vi "DriveModuleControl.vi"(8 "error in":errorcluster, 9 "Actual State":T1={"Speed"=0.0, "Angle"={"VALUE"=0.0, "COS"=1.0, "SIN"=0.0}} {"Angle"."SIN" format="%13.4f"; "Angle"."COS" format="%13.4f"; "Angle"."VALUE" format="%13.4f"}, 10 "Desired State":T1={"Speed"=0.0, "Angle"={"VALUE"=0.0, "COS"=1.0, "SIN"=0.0}} {"Angle"."SIN" format="%13.4f"; "Angle"."COS" format="%13.4f"; "Angle"."VALUE" format="%13.4f"}, 11 "ModualNamePrefix":i32) -> (0 "error out":errorcluster)   [LabVIEW 2023]
uses:
  <vilib>/Rock Robotics/WPI/ThirdParty/JAS_Junk/TrajLib/TypeDef/SWERVE_DRIVE_MODULE_STATE.ctl
  <vilib>/Rock Robotics/WPI/ThirdParty/JAS_Junk/TrajLib/TypeDef/ROTATION2D.ctl
  <vilib>/Rock Robotics/WPI/ThirdParty/JAS_Junk/TrajLib/Rotation2d_Minus.vi
  <vilib>/Rock Robotics/WPI/ThirdParty/JAS_Junk/TrajLib/Rotation2d_GetRadians.vi
  <vilib>/Rock Robotics/WPI/ThirdParty/JAS_Junk/TrajLib/SwerveModuleState_New.vi
  <vilib>/Rock Robotics/WPI/ThirdParty/JAS_Junk/TrajLib/Rotation2d_RotateBy.vi
  <vilib>/Rock Robotics/WPI/ThirdParty/JAS_Junk/TrajLib/Rotation2d_CreateAngle.vi
  <vilib>/Rock Robotics/WPI/ThirdParty/JAS_Junk/TrajLib/SimpleMotorFF_Calculate.vi
  <vilib>/Rock Robotics/WPI/ThirdParty/JAS_Junk/TrajLib/PIDController_AtSetpoint.vi
  <vilib>/Rock Robotics/WPI/ThirdParty/JAS_Junk/TrajLib/PIDController_SetPIDF.vi
  <vilib>/Rock Robotics/WPI/ThirdParty/JAS_Junk/TrajLib/PIDController_SetDerivativeFilter.vi
  <vilib>/Rock Robotics/WPI/ThirdParty/JAS_Junk/TrajLib/PIDController_SetIntegratorRange.vi
  <vilib>/Rock Robotics/WPI/ThirdParty/JAS_Junk/TrajLib/PIDController_SetTolerancePandV.vi
  <vilib>/Rock Robotics/WPI/ThirdParty/JAS_Junk/TrajLib/PIDController_DisableContinousInput.vi
  <vilib>/Rock Robotics/WPI/ThirdParty/JAS_Junk/TrajLib/PIDController_EnableContinousInput.vi
  <vilib>/Rock Robotics/WPI/ThirdParty/JAS_Junk/TrajLib/PIDController_Reset.vi
  <vilib>/Rock Robotics/WPI/ThirdParty/JAS_Junk/TrajLib/PIDController_New.vi
  <vilib>/Rock Robotics/WPI/ThirdParty/JAS_Junk/TrajLib/PIDController_SetOutputLimits.vi
  <vilib>/Rock Robotics/WPI/ThirdParty/JAS_Junk/TrajLib/VI/PIDController_SetIntegratorZone.vi
  <vilib>/Rock Robotics/WPI/ThirdParty/JAS_Junk/TrajLib/SlewRateLimiter_New.vi
  <vilib>/Rock Robotics/WPI/ThirdParty/JAS_Junk/TrajLib/SlewRateLimiter_Reset.vi
  <vilib>/Rock Robotics/WPI/ThirdParty/JAS_Junk/TrajLib/SlewRateLimiter_Calculate.vi
  <vilib>/Rock Robotics/WPI/ThirdParty/JAS_Junk/TrajLib/SlewRateLimiter_SetRate.vi
  <vilib>/Rock Robotics/WPI/ThirdParty/JAS_Junk/TrajLib/Rotation2d_UnaryMinus.vi
  <vilib>/Rock Robotics/WPI/ThirdParty/JAS_Junk/TrajLib/Rotation2d_CreateXY.vi
  <vilib>/Rock Robotics/WPI/ThirdParty/JAS_Junk/TrajLib/PIDController_NewPeriod.vi
  <vilib>/Rock Robotics/WPI/ThirdParty/JAS_Junk/TrajLib/Util_GetTime.vi
  <vilib>/Rock Robotics/WPI/ThirdParty/JAS_Junk/TrajLib/Util_CalcDist.vi
  <vilib>/Rock Robotics/SystemInterfaces/NetworkCommunication/NetComm_UsageReport_report.vi
  <vilib>/Rock Robotics/WPI/ThirdParty/JAS_Junk/TrajLib/VI/Util_GetTime_U32.vi
  DriveGlobal.vi
  <vilib>/Rock Robotics/SystemInterfaces/Utilities/FPGA_UtilitiesRead LocalTime.vi
  <vilib>/Rock Robotics/WPI/ThirdParty/JAS_Junk/TrajLib/VI/Util_GetTime_U64.vi
  <vilib>/Rock Robotics/WPI/ThirdParty/JAS_Junk/TrajLib/Globals/Util_LibraryGlobals.vi
  <vilib>/Rock Robotics/WPI/ThirdParty/JAS_Junk/TrajLib/PIDController_AdvCalculate_FF_Sp_Pv.vi
  <vilib>/Rock Robotics/Network Tables/NT Write Number.vi
  <vilib>/Rock Robotics/WPI/ThirdParty/JAS_Junk/TrajLib/Trajectory_Library.lvlib
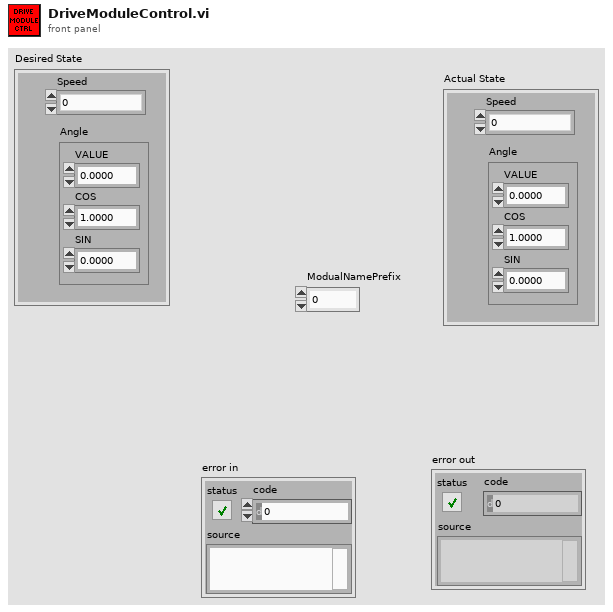
[diagram p1: front panel]
types:
  T1 = typedef "Trajectory_Library.lvlib/SWERVE_DRIVE_MODULE_STATE.ctl" = cluster{"Speed":dbl, "Angle":T2}
  T2 = typedef "Trajectory_Library.lvlib/ROTATION2D.ctl" = cluster{"VALUE":dbl, "COS":dbl, "SIN":dbl}
  T3 = typedef "Trajectory_Library.lvlib/SIMPLE_MOTOR_FF.ctl" = cluster{"Ks":dbl, "Kv":dbl, "Ka":dbl, "KnInv":dbl}
  T4 = typedef "Trajectory_Library.lvlib/PID_ADV_LIMITS.ctl" = cluster{"MaxInput":dbl, "MinInput":dbl, "Continuous":bool, "MaxOutput":dbl, "MinOutput":dbl}
  T5 = typedef "Trajectory_Library.lvlib/PID_ADV_TUNING.ctl" = cluster{"Kf":dbl, "Kp":dbl, "Ki":dbl, "Kd":dbl, "MaximumIntegral":dbl, "MinimumIntegral":dbl, "Filter Derivative":bool, "IntegralZone":dbl}
  T6 = typedef "WPI_MotorControlDeviceRef.ctl" = cluster{"DeviceStatus":errorcluster, "Type":T7, "PWM":cluster{"PWM Channel":T8, "DeadBand":T9}, "CAN":cluster{"Device Number":u8, "SetOutput VI Ref":variant, "GetOutput VI Ref":variant, "Enable VI Ref":variant, "Disable VI Ref":variant, "Data":variant}, "Invert":bool, "DIO PWM":cluster{"PWM \"Enable\" Channel":T8, "DIOChannel":T10, "PWM Rate":dbl}}
  T7 = typedef "WPI_MotorControlType.ctl" = enum16{"PWM", "CAN", "DIO PWM"}
  T8 = typedef "FPGA_DIOPWMChannel.ctl" = enum8{"PWM 0", "PWM 1", "PWM 2", "PWM 3", "PWM 4", "PWM 5", "PWM 6", "PWM 7", "PWM 8", "PWM 9", "PWM MXP 0", "PWM MXP 1", "PWM MXP 2", "PWM MXP 3", "PWM MXP 4", "PWM MXP 5", "PWM MXP 6", "PWM MXP 7", "PWM MXP 8", "PWM MXP 9", "Invalid"}
  T9 = typedef "WPI_PWMDeadband.ctl" = cluster{"Name":string, "maxPositivePwm":i32, "minPositivePwm":i32, "centerPwm":i32, "maxNegativePwm":i32, "minNegativePwm":i32, "angularRange":u16}
  T10 = typedef "FPGA_DIOChannel.ctl" = enum8{"DIO 0", "DIO 1", "DIO 2", "DIO 3", "DIO 4", "DIO 5", "DIO 6", "DIO 7", "DIO 8", "DIO 9", "DIO MXP 0", "DIO MXP 1", "DIO MXP 2", "DIO MXP 3", "DIO MXP 4", "DIO MXP 5", "DIO MXP 6", "DIO MXP 7", "DIO MXP 8", "DIO MXP 9", "DIO MXP 10", "DIO MXP 11", "DIO MXP 12", "DIO MXP 13", "DIO MXP 14", "DIO MXP 15", "SPI Port CS1", "SPI Port CS2", "SPI Port CS3", "SPI Port MISO", "SPI Port MOSI", "Invalid"}
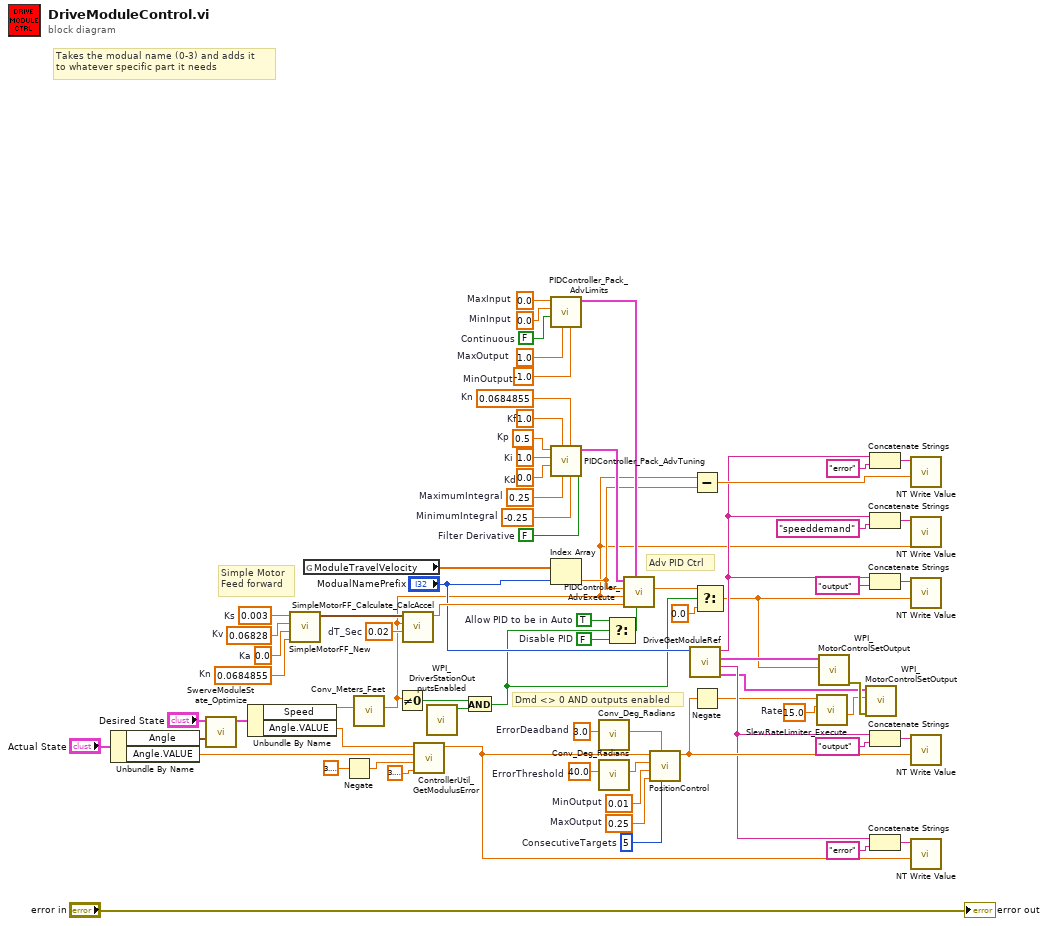
[diagram p0: block diagram]
diagram:
  w3 = 15.0  # Rate
  w4 = TRUE  # Allow PID to be in Auto
  w6 = FALSE  # Disable PID
  w19 = 0.0684855  # Kn
  w36 = 0.5  # Kp
  w35 = 1.0  # Ki
  w34 = 0.0  # Kd
  w33 = 1.0  # Kf
  w32 = 0.25  # MaximumIntegral
  w31 = -0.25  # MinimumIntegral
  w30 = FALSE  # Filter Derivative
  w28 = 0.0  # MinInput
  w27 = FALSE  # Continuous
  w26 = 1.0  # MaxOutput
  w29 = -1.0  # MinOutput
  w25 = 0.0  # MaxInput
  w46 = 0.0684855  # Kn
  w45 = 0.02  # dT_Sec
  w43 = 0.003  # Ks
  w42 = 0.06828  # Kv
  w41 = 0.0  # Ka
  w56 = 5  # ConsecutiveTargets
  w53 = 0.25  # MaxOutput
  w57 = 0.01  # MinOutput
  w50 = 40.0  # ErrorThreshold
  w52 = 3.0  # ErrorDeadband
  # "Dmd <> 0 AND outputs enabled"
  # "Adv PID Ctrl"
  # "Simple Motor\nFeed forward"
  # "Takes the modual name (0-3) and adds it \nto whatever specific part it needs"
  n1 = Unbundle By Name("Actual State") -> ("Angle"=w64:T2, "Angle.VALUE"=w60:dbl)
  n2 = call <vilib>:"SwerveModuleState_Optimize.vi"("CurrentAngle"=w64, "Desired State"="Desired State") -> ("out SWERVE_DRIVE_MODULE_STATE"=w62:T1)  [unwired: 9 in]
  n3 = Unbundle By Name(w62) -> ("Speed"=w47:dbl, "Angle.VALUE"=w61:dbl)
  n4 = call <vilib>:"SimpleMotorFF_New.vi"("Kn"=w46, "Ka"=w41, "Kv"=w42, "Ks"=w43) -> ("SIMPLE_MOTOR_FF"=w44:T3)  [unwired: 7 in]
  n5 = global read "DriveGlobal.vi" "ModuleTravelVelocity"() -> (w21:dbl[])
  n6 = Negate(x=3.141592653589793) -> (-x=w63:dbl)
  n7 = call <vilib>:"Conv_Meters_Feet.vi"("Meters"=w47) -> ("Feet"=w13:dbl)  [unwired: 10 in]
  n8 = Not Equal To 0?(x=w13) -> (x != 0?=w8:bool)
  n9 = call <vilib>:"SimpleMotorFF_Calculate_CalcAccel.vi"("dT_Sec"=w45, "VelSp"=w13, "SIMPLE_MOTOR_FF"=w44) -> ("FeedForward"=w22:dbl)  [unwired: 8 in]
  n10 = call <vilib>:"ControllerUtil_GetModulusError.vi"("Maximum_Input"=3.141592653589793, "Minimum_Input"=w63, "Measurerment(PV)"=w60, "Reference(SP)"=w61) -> ("Error"=w54:dbl)  [unwired: 7 in]
  n11 = call <vilib>:"WPI_DriverStationOutputsEnabled.vi"() -> ("OutputsEnabled?"=w9:bool)  [unwired: 10 in, 1 out]
  n12 = And(x=w8, y=w9) -> (x .and. y?=w5:bool)
  n13 = call <vilib>:"PIDController_Pack_AdvLimits.vi"("MinOutput"=w29, "MaxOutput"=w26, "Continuous"=w27, "MinInput"=w28, "MaxInput"=w25) -> ("Adv PID Limits"=w23:T4)  [unwired: 6 in]
  n14 = call <vilib>:"PIDController_Pack_AdvTuning.vi"("Filter Derivative"=w30, "MinimumIntegral"=w31, "Kn"=w19, "MaximumIntegral"=w32, "Kf"=w33, "Kd"=w34, "Ki"=w35, "Kp"=w36) -> ("Adv PID Tuning"=w24:T5)  [unwired: 3 in]
  n15 = Index Array(array=w21, index="ModualNamePrefix") -> (element=w18:dbl)
  n16 = call <vilib>:"Conv_Deg_Radians.vi"("Degress"=w52) -> ("Radians"=w51:dbl)  [unwired: 10 in]
  n17 = call <vilib>:"Conv_Deg_Radians.vi"("Degress"=w50) -> ("Radians"=w49:dbl)  [unwired: 10 in]
  n18 = Select(t=w4, s=w5, f=w6) -> (s? t:f=w7:bool)
  n19 = call <vilib>:"PIDController_AdvExecute.vi"("Auto"=w7, "Adv PID Limits"=w23, "FF-FeedForward"=w22, "SP-SetPoint"=w13, "PV-Measurement"=w18, "Adv PID Tuning"=w24) -> ("CO-ControlOutput"=w11:dbl)  [unwired: 3 in, 2 out]
  n20 = call "PositionControl.vi"("ConsecutiveTargets"=w56, "ErrorDeadband"=w51, "MaxOutput"=w53, "MinOutput"=w57, "ErrorThreshold"=w49, "Error"=w54) -> ("OutputValue"=w48:dbl)  [unwired: 3 in, 2 out]
  n21 = call "DriveGetModuleRef.vi"("ModualNamePrefix"="ModualNamePrefix") -> ("SpinMot"=w37:T6, "SpinStr"=w38:string, "TravMot"=w39:T6, "TravStr"=w14:string)  [unwired: 5 in, 2 out]
  n22 = Subtract(x=w13, y=w18) -> (x-y=w15:dbl)
  n23 = Negate(x=w48) -> (-x=w2:dbl)
  n24 = Select(t=w11, s=w5, f=0.0 ("t")) -> (s? t:f=w12:dbl)
  n25 = call <vilib>:"SlewRateLimiter_Execute.vi"("PositiveRate"=w3, "Input"=w2) -> ("Output"=w1:dbl)  [unwired: 8 in, 1 out]
  n26 = call <vilib>:"WPI_MotorControlSetOutput.vi"("Output"=w12, "MotorControlDevRef"=w39) -> ("error out"=w40:errorcluster)  [unwired: 7 in, 2 out]
  n27 = call <vilib>:"WPI_MotorControlSetOutput.vi"("error in (no error)"=w40, "Output"=w1, "MotorControlDevRef"=w37) -> ()  [unwired: 6 in, 3 out]
  n28 = Concatenate Strings(w14, "error" ("refnum name")) -> (w16:string)
  n29 = Concatenate Strings(w14, "speeddemand" ("refnum name")) -> (w72:string)
  n30 = Concatenate Strings(w14, "output" ("refnum name")) -> (w70:string)
  n31 = Concatenate Strings(w38, "output" ("refnum name")) -> (w55:string)
  n32 = Concatenate Strings(w38, "error" ("refnum name")) -> (w68:string)
  n33 = call-poly <vilib>:"NT Write Value.vi"("value"=w15, "name"=w16) -> ()  [unwired: 9 in, 1 out]
  n34 = call-poly <vilib>:"NT Write Value.vi"("value"=w13, "name"=w72) -> ()  [unwired: 9 in, 1 out]
  n35 = call-poly <vilib>:"NT Write Value.vi"("value"=w12, "name"=w70) -> ()  [unwired: 9 in, 1 out]
  n36 = call-poly <vilib>:"NT Write Value.vi"("value"=w48, "name"=w55) -> ()  [unwired: 9 in, 1 out]
  n37 = call-poly <vilib>:"NT Write Value.vi"("value"=w54, "name"=w68) -> ()  [unwired: 9 in, 1 out]
  "error out" <- "error in"
